vi "CSV_ConditionalDataCheck.vi"(7 "Headers":string[](array[string])=["Numeric Data", "String Data"], 8 "error in":errorcluster, 9 "A[StringData]":string[](array[string])=["401", "q"], 10 "A[StringLabels]":string[](array[string])=["Numeric Data", "String Data"], 11 "Data":string="Numeric Data,Float Data,String Data,Enum Data,Array Data[0].Numeric Data\n100,100.123000,'This is string','Enum Item 2',1\nNumeric Data,Float Data,String Data,Enum Data,Array Data[0].Numeric Data,Array Data[1].Numeric Data\n100,100.123000,'This is string','Enum Item 2',1,2\n100,100.123000,'This is string','Enum Item 2',1,3\n100,100.123000,'This is string','Enum Item 2',1,2\n100,100.123000,'This is string','Enum Item 2',1,2\nNumeric Data,Float Data,String Data,Enum Data,Array Data[0].Numeric Data,Array Data[1].Numeric Data,Array Data[2].Numeric Data\n100,100.123000,'This is string','Enum Item 2',1,2,3\n100,100.123000,'This is string','Enum Item 2',1,2,3\n100,100.123000,'This is string','Enum Item 2',1,45,6\nNumeric Data,Float Data,String Data,Enum Data,Array Data[0].Numeric Data,Array Data[1].Numeric Data\n100,100.123000,'This is string','Enum Item 2',1,5\n100,100.123000,'This is string','Enum Item 2',1,8\nNumeric Data,Float Data,String Data,Enum Data,Array Data[0].Numeric Data,Array Data[1].Numeric Data,Array Data[2].Numeric Data,Array Data[3].Numeric Data\n401,100.123000,'q','Enum Item 2',1,0,0,5\nNumeric Data,Float Data,String Data,Enum Data,Array Data[0].Numeric Data\n100,100.123000,'This is string','Enum Item 2',1\n100,100.123000,'This is string','Enum Item 2',18\nNumeric Data,Float Data,String Data,Enum Data,Array Data[0].Numeric Data,Array Data[1].Numeric Data,Array Data[2].Numeric Data,Array Data[3].Numeric Data,Array Data[4].Numeric Data\n100,100.123000,'This is string','Enum Item 2',1,0,0,0,98\nNumeric Data,Float Data,String Data,Enum Data,Array Data[0].Numeric Data,Array Data[1].Numeric Data\n100,100.123000,'This is string','Enum Item 2',1,2\nNumeric Data,Float Data,String Data,Enum Data,Array Data[0].Numeric Data,Array Data[1].Numeric Data,Array Data[2].Numeric Data\n100,100.123000,'This is string','Enum Item 2',1,2,2\nNumeric Data,Float Data,String Data,Enum Data,Array Data[0].Numeric Data\n100,100.123000,'This is string','Enum Item 2',1\n") -> (0 "error out":errorcluster, 1 "Selected Headers":string[][](array[string]), 2 "Indexes for Conditional Data":i32[](array[numeric]), 3 "Data in 2D":string[][](array[string]), 4 "Seleted Indices":i32[](array[numeric]))   [LabVIEW 2014, in "TableLogger_CSV_Actor.lvlib" / "TableLogger_CSV_Actor.lvclass"]
uses:
  TableLogger_CSV_Actor.lvclass
  <userlib>/_OpenG.lib/array/array.llb/Search 1D Array (String)__ogtk.vi
  <userlib>/_OpenG.lib/array/array.llb/Search 1D Array (I32)__ogtk.vi
  <userlib>/_OpenG.lib/array/array.llb/Delete Elements from 1D Array (I32)__ogtk.vi
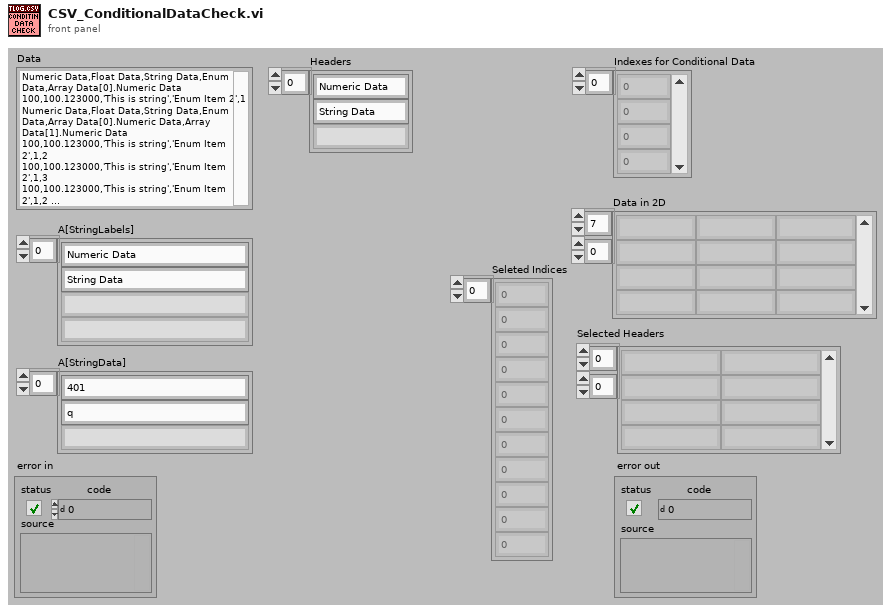
[diagram p1: front panel]
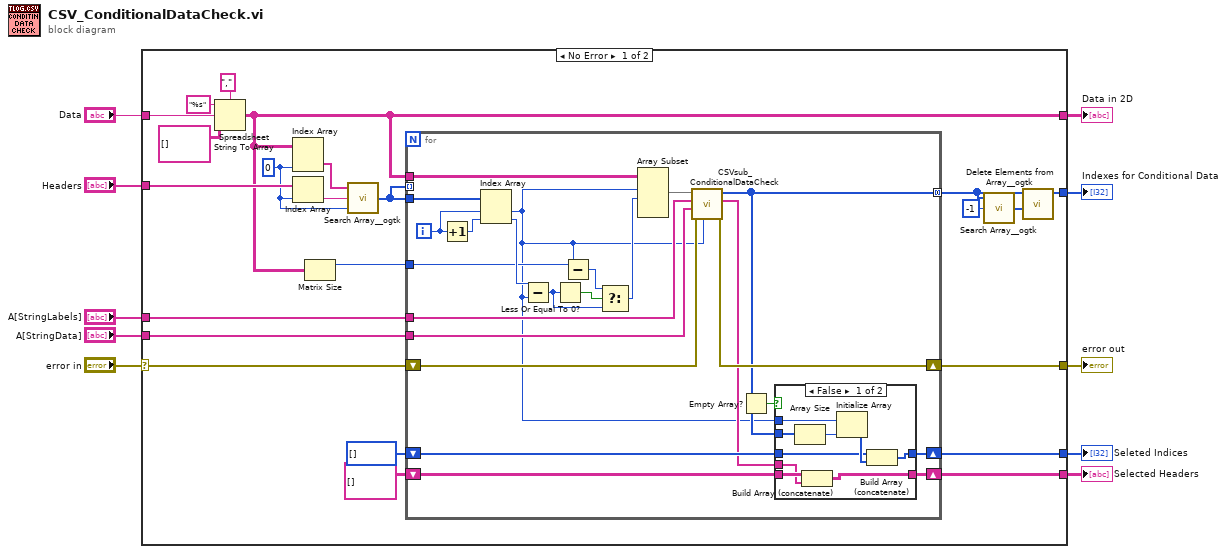
[diagram p0: block diagram]
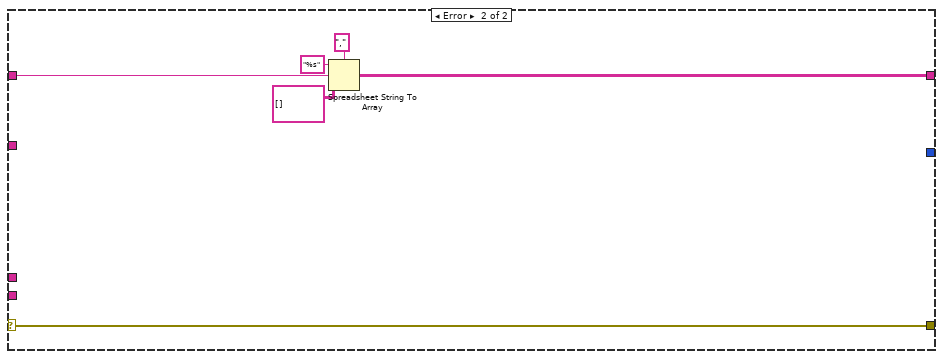
[diagram p3: hidden frame]
diagram:
  n1 = case shown="No Error" "error in" {
    selector: "error in" -> [w32 w73]
    tunnel: [w17 w68] -> w4
    tunnel: [w24 _] -> w5
    tunnel: [w33 w73] -> w10
    tunnel: "A[StringLabels]" -> [w31 _]
    tunnel: "A[StringData]" -> [w30 _]
    tunnel: "Data" -> [w18 w69]
    tunnel: "Headers" -> [w23 _]
    tunnel: [w12 _] -> w1
    tunnel: [w11 _] -> w2
    frame No Error {
      w15 = 0 ("disabled index (col)")
      n2 = Spreadsheet String To Array(delimiter (Tab)=",", format string="%s", spreadsheet string=w18, array type (2D Dbl)=string[][] []) -> (array=w17:string[][])
      n3 = Index Array(array=w17, index (col)=w15) -> (element=w16:string[])  [unwired: 1 in]
      n4 = Index Array(array=w23, index=w15) -> (element=w22:string)
      n5 = Matrix Size(0:w17) -> (1:w28:i32)  [unwired: 1 out]
      n6 = call-poly <userlib>:"Search Array__ogtk.vi"("Array"=w16, "Element Data"=w22, "Start Index (0)"=w15) -> ("Indices of Elements"=w29:i32[])  [unwired: 6 in]
      n7 = for {
        tunnel: [w41] -> w25 mode=concatenating
        shift-right: [w50] -> w33
        shift-left: w32 -> [w51]
        tunnel: w29 -> [w56]
        tunnel: w17 -> [w45]
        tunnel: w31 -> [w53]
        tunnel: w30 -> [w52]
        tunnel: w29 -> [_] mode=indexing
        tunnel: w28 -> [w44]
        shift-right: [w39] -> w12
        shift-left: i32[] [] -> [w38]
        shift-right: [w37] -> w11
        shift-left: string[][] [] -> [w35]
        i -> [w42]
        n8 = Increment(x=w42) -> (x+1=w54:i32)
        n9 = Index Array(array=w56, index #1=w42, index #2=w54) -> (element #1=w34:i32, element #2=w55:i32)
        n10 = Subtract(x=w55, y=w34) -> (x-y=w46:i32)
        n11 = Less Or Equal To 0?(x=w46) -> (x <= 0?=w48:bool)
        n12 = Subtract(x=w44, y=w34) -> (x-y=w43:i32)
        n13 = Select(t=w43, s=w48, f=w46) -> (s? t:f=w47:i32)
        n14 = Array Subset(array=w45, index (row)=w34, length (row)=w47) -> (w49:string[][])  [unwired: 2 in]
        n15 = call "CSVsub_ConditionalDataCheck.vi"("index in"=w34, "error in"=w51, "A[StringData]"=w52, "A[StringLabels]"=w53, "Data"=w49) -> ("error out"=w50:errorcluster, "Headers"=w36:string[], "Data Index"=w41:i32[])  [unwired: 4 in]
        n16 = Empty Array?(array=w41) -> (empty?=w40:bool)
        n17 = case shown="False" w40 {
          tunnel: w34 -> [w65 _]
          tunnel: w41 -> [w63 _]
          tunnel: [w61 w67] -> w39
          tunnel: w38 -> [w60 w67]
          tunnel: [w57 w66] -> w37
          tunnel: w36 -> [w58 _]
          tunnel: w35 -> [w59 w66]
          frame False {
            n18 = Array Size(array=w63) -> (size(s)=w64:i32)
            n19 = Build Array (concatenate)(w59, w58) -> (w57:string[][])
            n20 = Initialize Array(w65, w64) -> (w62:i32[])
            n21 = Build Array (concatenate)(w60, w62) -> (w61:i32[])
          }
          frame True {
          }
        }
      }
      n22 = call-poly <userlib>:"Search Array__ogtk.vi"("Array"=w25, "Element Data"=-1) -> ("Indices of Elements"=w27:i32[])  [unwired: 7 in]
      n23 = call-poly <userlib>:"Delete Elements from Array__ogtk.vi"("indices"=w27, "array"=w25) -> ("array w/ subset deleted"=w24:i32[])  [unwired: 8 in, 1 out]
    }
    frame Error {
      n24 = Spreadsheet String To Array(delimiter (Tab)=",", format string="%s", spreadsheet string=w69, array type (2D Dbl)=string[][] []) -> (array=w68:string[][])
    }
  }
  "Data in 2D" <- w4
  "Indexes for Conditional Data" <- w5
  "error out" <- w10
  "Selected Headers" <- w2
  "Seleted Indices" <- w1
